vi "Periodic Tasks.vi"(8 "error in":errorcluster) -> ()   [LabVIEW 2023]
doc: "This VI runs in parallel to other tasks. It can contain as many user-defined periodic loops as you need. These can carry out PID or other sorts of timed response."
uses:
  <vilib>/Rock Robotics/WPI/Utilities/WPI_GetSetVariantRefNum.vi
  <vilib>/Rock Robotics/WPI/Ultrasonic/WPI_SonarSRF04DigitalRefNum Registry Get.vi
  <vilib>/Rock Robotics/Network Tables/NT Read Number.vi
  Robot Global Data.vi
  <vilib>/Rock Robotics/Network Tables/NT Write Number.vi
  <vilib>/Rock Robotics/WPI/Ultrasonic/WPI_SonarSRF04DigitalGetRange.vi
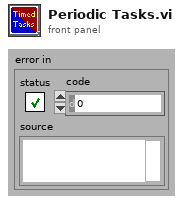
[diagram p1: front panel]
types:
  T1 = typedef "WPI_JoystickDevRef.ctl" = cluster{"Device":T2}
  T2 = typedef "WPI_JoystickDeviceEnum.ctl" = enum16{"USB 0", "USB 1", "USB 2", "USB 3", "USB 4", "USB 5"}
  T3 = typedef "WPI_RobotDriveDevRef.ctl" = cluster{"DevStatus":errorcluster, "Motors[]":T4[], "Square Inputs":bool, "Max Output":dbl}
  T4 = typedef "WPI_MotorControlDeviceRef.ctl" = cluster{"DeviceStatus":errorcluster, "Type":T5, "PWM":cluster{"PWM Channel":T6, "DeadBand":T7}, "CAN":cluster{"Device Number":u8, "SetOutput VI Ref":variant, "GetOutput VI Ref":variant, "Enable VI Ref":variant, "Disable VI Ref":variant, "Data":variant}, "Invert":bool, "DIO PWM":cluster{"PWM \"Enable\" Channel":T6, "DIOChannel":T8, "PWM Rate":dbl}}
  T5 = typedef "WPI_MotorControlType.ctl" = enum16{"PWM", "CAN", "DIO PWM"}
  T6 = typedef "FPGA_DIOPWMChannel.ctl" = enum8{"PWM 0", "PWM 1", "PWM 2", "PWM 3", "PWM 4", "PWM 5", "PWM 6", "PWM 7", "PWM 8", "PWM 9", "PWM MXP 0", "PWM MXP 1", "PWM MXP 2", "PWM MXP 3", "PWM MXP 4", "PWM MXP 5", "PWM MXP 6", "PWM MXP 7", "PWM MXP 8", "PWM MXP 9", "Invalid"}
  T7 = typedef "WPI_PWMDeadband.ctl" = cluster{"Name":string, "maxPositivePwm":i32, "minPositivePwm":i32, "centerPwm":i32, "maxNegativePwm":i32, "minNegativePwm":i32, "angularRange":u16}
  T8 = typedef "FPGA_DIOChannel.ctl" = enum8{"DIO 0", "DIO 1", "DIO 2", "DIO 3", "DIO 4", "DIO 5", "DIO 6", "DIO 7", "DIO 8", "DIO 9", "DIO MXP 0", "DIO MXP 1", "DIO MXP 2", "DIO MXP 3", "DIO MXP 4", "DIO MXP 5", "DIO MXP 6", "DIO MXP 7", "DIO MXP 8", "DIO MXP 9", "DIO MXP 10", "DIO MXP 11", "DIO MXP 12", "DIO MXP 13", "DIO MXP 14", "DIO MXP 15", "SPI Port CS1", "SPI Port CS2", "SPI Port CS3", "SPI Port MISO", "SPI Port MOSI", "Invalid"}
  T9 = typedef "WPI_UltrasonicDeviceRef.ctl" = cluster{"DevStatus":errorcluster, "Ping Channel":T8, "Echo Channel":T8, "CntIndex":T10}
  T10 = typedef "FPGA_CounterCtrSystemIndex.ctl" = enum8{"Ctr 0", "Ctr 1", "Ctr 2", "Ctr 3", "Ctr 4", "Ctr 5", "Ctr 6", "Ctr 7", "Invalid"}
  T11 = typedef "WPI_GyroDevRef.ctl" = cluster{"DevStatus":errorcluster, "Analog Channel":T12, "Gain (VoltsPerDegree/Second)":dbl, "Gyro Type":enum16{"Analog", "XRS450"}, "Handle":i32, "SPI Bus":T13, "Device Found":bool, "Sample Rate":dbl, "Calibrate On Open":bool, "Offset":dbl}
  T12 = typedef "FPGA_AIChannel.ctl" = enum8{"AI 0", "AI 1", "AI 2", "AI 3", "AI MXP 0", "AI MXP 1", "AI MXP 2", "AI MXP 3", "Invalid"}
  T13 = typedef "spi_bus.ctl" = enum16{"SPI On-Board, CS0", "SPI On-Board, CS1", "SPI On-Board, CS2", "SPI On-Board, CS3", "SPI MXP", "Invalid"}
  T14 = cluster{"JoystickDevRef":T1, "RobotDriveDevRef":T3}
  T15 = typedef "WPI_ServoDeviceRef.ctl" = cluster{"DeviceStatus":errorcluster, "PWM Channel":T6, "DeadBand":T7}
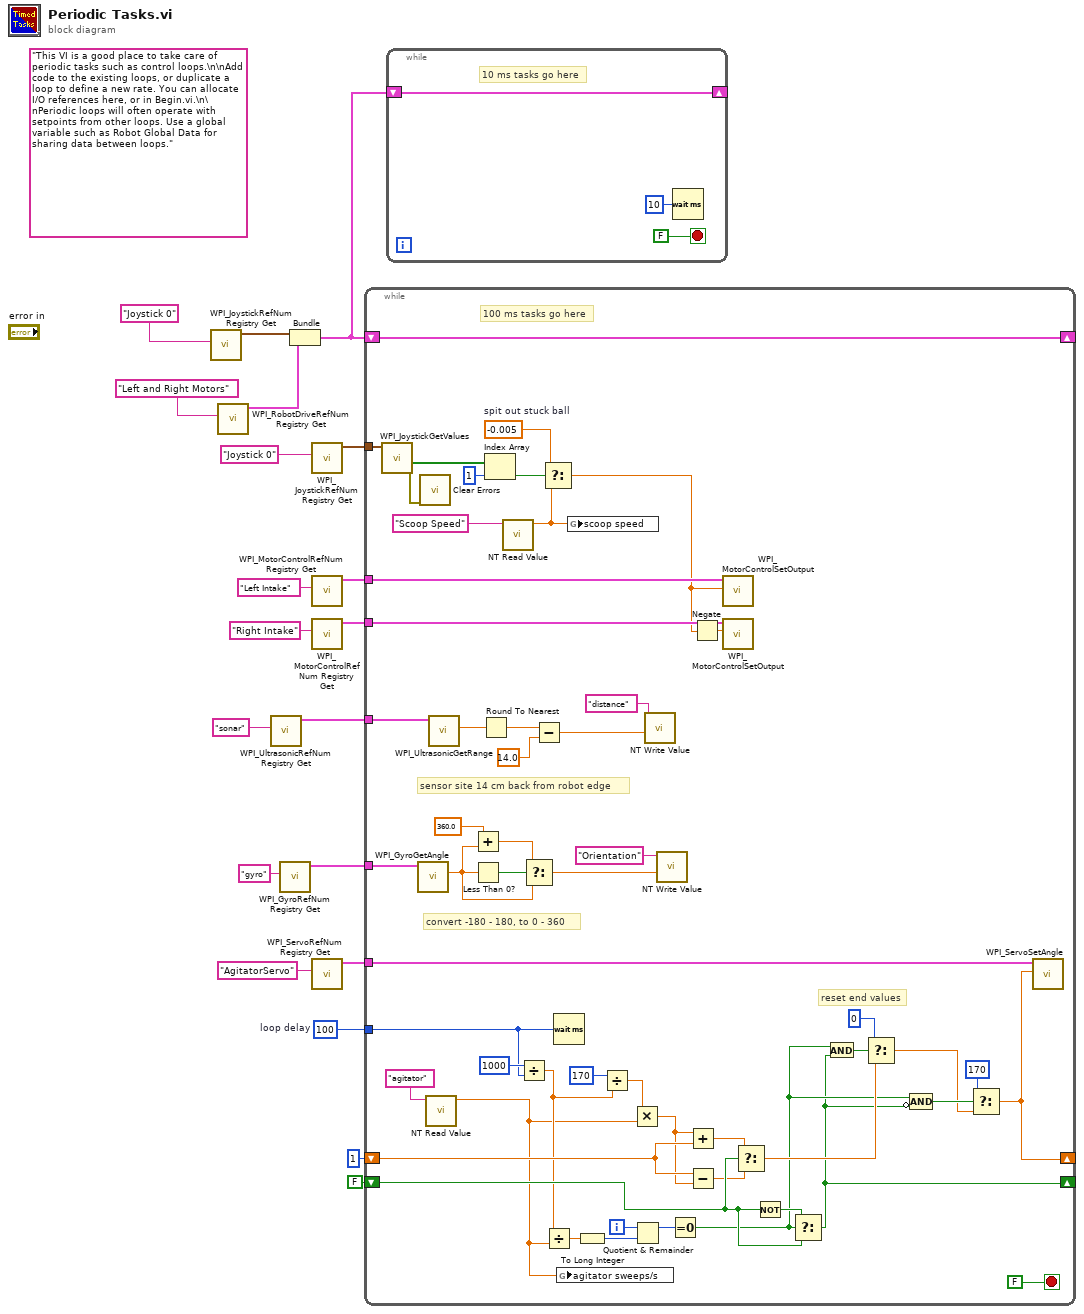
[diagram p0: block diagram]
diagram:
  w5 = u32 100  # loop delay
  (unwired) "This VI is a good place to take care of periodic tasks such as control loops.\n\nAdd code to the existing loops, or duplicate a loop to define a new rate. You can allocate I/O references here, or in Begin.vi.\n\nPeriodic loops will often operate with setpoints from other loops. Use a global variable such as Robot Global Data for sharing data between loops."
  n1 = call <vilib>:"WPI_JoystickRefNum Registry Get.vi"("refnum name"="Joystick 0") -> ("JoystickDevRef"=w18:T1)  [unwired: 1 in, 9 out]
  n2 = call <vilib>:"WPI_RobotDriveRefNum Registry Get.vi"("refnum name"="Left and Right Motors") -> ("RobotDriveDevRef"=w17:T3)  [unwired: 1 in, 9 out]
  n3 = call-poly <vilib>:"WPI_UltrasonicRefNum Registry Get.vi"("refnum name"="sonar") -> ("SonarSRF04DevRef"=w3:T9)  [unwired: 9 in, 1 out]
  n4 = call <vilib>:"WPI_GyroRefNum Registry Get.vi"("refnum name"="gyro") -> ("GyroDevRef"=w1:T11)  [unwired: 9 in, 1 out]
  n5 = Bundle("JoystickDevRef"=w18, "RobotDriveDevRef"=w17) -> (w16:T14)  [unwired: 1 out]
  n6 = call <vilib>:"WPI_JoystickRefNum Registry Get.vi"("refnum name"="Joystick 0") -> ("JoystickDevRef"=w6:T1)  [unwired: 1 in, 9 out]
  n7 = call <vilib>:"WPI_MotorControlRefNum Registry Get.vi"("refnum name"="Left Intake") -> ("MotorControlDevRef"=w11:T4)  [unwired: 9 in, 1 out]
  n8 = call <vilib>:"WPI_MotorControlRefNum Registry Get.vi"("refnum name"="Right Intake") -> ("MotorControlDevRef"=w8:T4)  [unwired: 9 in, 1 out]
  n9 = call <vilib>:"WPI_ServoRefNum Registry Get.vi"("refnum name"="AgitatorServo") -> ("ServoDeviceRef"=w14:T15)  [unwired: 9 in, 1 out]
  n10 = while {
    shift-right: [w73] -> _
    shift-left: w16 -> [w73]
    tunnel: w14 -> [w72]
    shift-right: [w40] -> _
    shift-left: 1 ("Angle") -> [w54]
    shift-right: [w43] -> _
    shift-left: FALSE -> [w59]
    tunnel: w11 -> [w68]
    tunnel: w8 -> [w67]
    tunnel: w6 -> [w65]
    tunnel: w5 -> [w56]
    tunnel: w3 -> [w36]
    tunnel: w1 -> [w30]
    i -> [w71]
    stop <- FALSE stop-if-true
    w60 = -0.005  # spit out stuck ball
    # "convert -180 - 180, to 0 - 360"
    # "sensor site 14 cm back from robot edge"
    # "reset end values"
    # "100 ms tasks go here"
    n11 = call <vilib>:"WPI_JoystickGetValues.vi"("JoystickDevRef"=w65) -> ("error out"=w21:errorcluster, "Buttons"=w64:bool[])  [unwired: 6 in, 3 out]
    n12 = call <vilib>:"WPI_GyroGetAngle.vi"("GyroDevRef"=w30) -> ("Angle"=w25:dbl)  [unwired: 6 in, 4 out]
    n13 = call <vilib>:"Clear Errors.vi"("error in (no error)"=w21) -> ()  [unwired: 5 in, 2 out]
    n14 = call-poly <vilib>:"NT Read Value.vi"("name"="agitator" ("Name")) -> ("value"=w22:dbl)  [unwired: 8 in, 2 out]
    n15 = call-poly <vilib>:"WPI_UltrasonicGetRange.vi"("UltrasonicDevRef"=w36) -> ("Distance"=w35:dbl)  [unwired: 8 in, 2 out]
    n16 = Add(x=360.0, y=w25) -> (x+y=w26:dbl)
    n17 = Less Than 0?(x=w25) -> (x < 0?=w28:bool)
    n18 = Round To Nearest(number=w35) -> (nearest integer value=w33:dbl)
    n19 = Index Array(array=w64, index=1) -> (element=w62:bool)
    n20 = call-poly <vilib>:"NT Read Value.vi"("name"="Scoop Speed" ("Name")) -> ("value"=w37:dbl)  [unwired: 8 in, 2 out]
    n21 = Divide(x=u32 1000 ("loop delay"), y=w56) -> (x/y=w52:dbl)
    n22 = Select(t=w26, s=w28, f=w25) -> (s? t:f=w27:dbl)
    n23 = Subtract(x=w33, y=14.0) -> (x-y=w32:dbl)
    n24 = Select(t=w60, s=w62, f=w37) -> (s? t:f=w61:dbl)
    n25 = Divide(x=w52, y=w22) -> (x/y=w50:dbl)
    n26 = Wait (ms)(milliseconds to wait=w56) -> ()  [unwired: 1 out]
    n27 = global write "Robot Global Data.vi" "agitator sweeps/s"(w22) -> ()
    n28 = global write "Robot Global Data.vi" "scoop speed"(w37) -> ()
    n29 = To Long Integer(number=w50) -> (32bit integer=w48:i32)
    n30 = Divide(x=170 ("y"), y=w52) -> (x/y=w51:dbl)
    n31 = Multiply(x=w51, y=w22) -> (x*y=w49:dbl)
    n32 = Quotient & Remainder(x=w71, y=w48) -> (x-y*floor(x/y)=w70:i32)  [unwired: 1 out]
    n33 = call-poly <vilib>:"NT Write Value.vi"("value"=w32, "name"="distance" ("Name")) -> ()  [unwired: 9 in, 1 out]
    n34 = call-poly <vilib>:"NT Write Value.vi"("value"=w27, "name"="Orientation" ("Name")) -> ()  [unwired: 9 in, 1 out]
    n35 = Equal To 0?(x=w70) -> (x = 0?=w44:bool)
    n36 = Add(x=w49, y=w54) -> (x+y=w55:dbl)
    n37 = Subtract(x=w54, y=w49) -> (x-y=w58:dbl)
    n38 = Negate(x=w61) -> (-x=w66:dbl)
    n39 = call <vilib>:"WPI_MotorControlSetOutput.vi"("Output"=w61, "MotorControlDevRef"=w68) -> ()  [unwired: 7 in, 3 out]
    n40 = call <vilib>:"WPI_MotorControlSetOutput.vi"("Output"=w66, "MotorControlDevRef"=w67) -> ()  [unwired: 7 in, 3 out]
    n41 = Select(t=w55, s=w59, f=w58) -> (s? t:f=w45:dbl)
    n42 = Not(x=w59) -> (.not. x?=w69:bool)
    n43 = Select(t=w69, s=w44, f=w59) -> (s? t:f=w43:bool)
    n44 = And(x=w44, y=w43) -> (x .and. y?=w47:bool)
    n45 = Select(t=0 ("y"), s=w47, f=w45) -> (s? t:f=w41:dbl)
    n46 = Compound Arithmetic op=AND(w44, invert w43) -> (w42:bool)
    n47 = Select(t=170 ("y"), s=w42, f=w41) -> (s? t:f=w40:dbl)
    n48 = call <vilib>:"WPI_ServoSetAngle.vi"("Angle"=w40, "ServoDeviceRef"=w72) -> ()  [unwired: 8 in, 2 out]
  }
  n49 = while {
    shift-right: [w75] -> _
    shift-left: w16 -> [w75]
    stop <- FALSE stop-if-true
    # "10 ms tasks go here"
    n50 = Wait (ms)(milliseconds to wait=u32 10) -> ()  [unwired: 1 out]
  }
